vi "simulation de l ASSIETTE.vi"() -> ()   [LabVIEW 2016]
uses:
  <vilib>/Utility/miscctls.llb/LV3DPointTypeDef.ctl
  <vilib>/Instr/_visa.llb/VISA Configure Serial Port (Instr).vi
panel:
  in  "?":enum32{"Vue de l'ensemble"}(tab)
  out "2 2":dynamicdata(graph)
  in  "Aileron":dbl(slide) scale=-25.0..25.0
  out "Gimbal":refnum<vi>(3d-picture)
  in  "PITCH":dbl(slide) scale=-90.0..90.0
  in  "Profondeur":dbl(slide) scale=-35.0..35.0
  out "GAZ":dbl(slide) scale=0.0..35.0
  out "?":T1(graph)={"X"=[{"Y"=[21.620706805998168, 20.15124367946963, 12.465582235692763, 7.946576972490323, 11.656565240893995, 3.970903792227472, 5.440366929130449, 13.126028372052978, 19.003880895383112, 16.244982298473555, 16.832767550897515, 24.922937499080067, 24.33515224168201, 19.81289788882929, 13.93504536742159, 21.620706805998168], "Y"=[7.099604990531346, 5.077062500919932, 10.661022401488875, 5.291796067500631, 11.248807654089271, 16.832767550897515, 18.855310035128806, 13.271350139939326, 21.36152008350073, 25.220079209877188, 26.02909620777253, 20.151243679469633, 19.34222668734553, 20.773734831883043, 12.683564887248515, 7.099604990531346]}], "z"=[{"Y"=[15.0, 16.30733614, 17.60472267, 17.43107449, 17.60472267, 18.88228568, 20.13030215, 19.78828201, 20.13030215, 21.33927393, 22.5, 22.0, 22.5, 23.60364655, 24.64181415, 23.99902654, 24.64181415, 25.60660172, 26.49066665, 25.7246222, 26.49066665, 27.28728066, 27.99038106, 27.12435565, 27.99038106, 28.59461681, 29.09538931, 28.15569669, 29.09538931, 29.48888739, 29.7721163, 28.78730854, 29.7721163, 29.94292047, 30.0, 28.5, 30.0, 29.94292047, 29.7721163, 28.78730854, 29.7721163, 29.48888739, 29.09538931, 28.15569669, 29.09538931, 28.59461681, 27.99038106, 27.12435565, 27.99038106, 27.28728066, 26.49066665, 25.7246222, 26.49066665, 25.60660172, 24.64181415, 23.99902654, 24.64181415, 23.60364655, 22.5, 22.0, 22.5, 21.33927393, 20.13030215, 19.78828201, 20.13030215, 18.88228568, 17.60472267, 17.43107449, 17.60472267, 16.30733614, 15.0, 15.0, 15.0, 13.69266386, 12.39527733, 12.56892551, 12.39527733, 11.11771432, 9.86969785, 10.21171799, 9.86969785, 8.660726074, 7.5, 8.0, 7.5, 6.396353455, 5.358185855, 6.000973464, 5.358185855, 4.393398282, 3.509333353, 4.275377796, 3.509333353, 2.712719336, 2.009618943, 2.875644347, 2.009618943, 1.405383194, 0.904610688, 1.844303309, 0.904610688, 0.511112606, 0.227883705, 1.212691458, 0.227883705, 0.057079529, 0.0, 1.5, 0.0, 0.057079529, 0.227883705, 1.212691458, 0.227883705, 0.511112606, 0.904610688, 1.844303309, 0.904610688, 1.405383194, 2.009618943, 2.875644347, 2.009618943, 2.712719336, 3.509333353, 4.275377796, 3.509333353, 4.393398282, 5.358185855, 6.000973464, 5.358185855, 6.396353455, 7.5, 8.0, 7.5, 8.660726074, 9.86969785, 10.21171799, 9.86969785, 11.11771432, 12.39527733, 12.56892551, 12.39527733, 13.69266386, 15.0, 15.0], "Y"=[30.0, 29.94292047, 29.7721163, 28.78730854, 29.7721163, 29.48888739, 29.09538931, 28.15569669, 29.09538931, 28.59461681, 27.99038106, 27.12435565, 27.99038106, 27.28728066, 26.49066665, 25.7246222, 26.49066665, 25.60660172, 24.64181415, 23.99902654, 24.64181415, 23.60364655, 22.5, 22.0, 22.5, 21.33927393, 20.13030215, 19.78828201, 20.13030215, 18.88228568, 17.60472267, 17.43107449, 17.60472267, 16.30733614, 15.0, 15.0, 15.0, 13.69266386, 12.39527733, 12.56892551, 12.39527733, 11.11771432, 9.86969785, 10.21171799, 9.86969785, 8.660726074, 7.5, 8.0, 7.5, 6.396353455, 5.358185855, 6.000973464, 5.358185855, 4.393398282, 3.509333353, 4.275377796, 3.509333353, 2.712719336, 2.009618943, 2.875644347, 2.009618943, 1.405383194, 0.904610688, 1.844303309, 0.904610688, 0.511112606, 0.227883705, 1.212691458, 0.227883705, 0.057079529, 0.0, 1.5, 0.0, 0.057079529, 0.227883705, 1.212691458, 0.227883705, 0.511112606, 0.904610688, 1.844303309, 0.904610688, 1.405383194, 2.009618943, 2.875644347, 2.009618943, 2.712719336, 3.509333353, 4.275377796, 3.509333353, 4.393398282, 5.358185855, 6.000973464, 5.358185855, 6.396353455, 7.5, 8.0, 7.5, 8.660726074, 9.86969785, 10.21171799, 9.86969785, 11.11771432, 12.39527733, 12.56892551, 12.39527733, 13.69266386, 15.0, 15.0, 15.0, 16.30733614, 17.60472267, 17.43107449, 17.60472267, 18.88228568, 20.13030215, 19.78828201, 20.13030215, 21.33927393, 22.5, 22.0, 22.5, 23.60364655, 24.64181415, 23.99902654, 24.64181415, 25.60660172, 26.49066665, 25.7246222, 26.49066665, 27.28728066, 27.99038106, 27.12435565, 27.99038106, 28.59461681, 29.09538931, 28.15569669, 29.09538931, 29.48888739, 29.7721163, 28.78730854, 29.7721163, 29.94292047, 30.0, 28.5]}]}
  in  "ROLL":dbl(slide) scale=-90.0..90.0
  in  "Directions":dbl(slide) scale=-25.0..25.0
  in  "visual":refnum<k7>(container) caption="3D 파라미터형 표면"
  out "2":dynamicdata(graph)
  out "Temperature":dbl caption="degC" format="%.1f"
  out "Altitude Estimée":dbl caption="m" format="%.1f"
  in  "VISA resource name":refnum<visa-resource-name>
  in  "yaw":dbl(slide) scale=0.0..360.0
  in  "stop":bool
  in  "Heading":dbl(knob) scale=-360.0..360.0
  out "?":timestamp
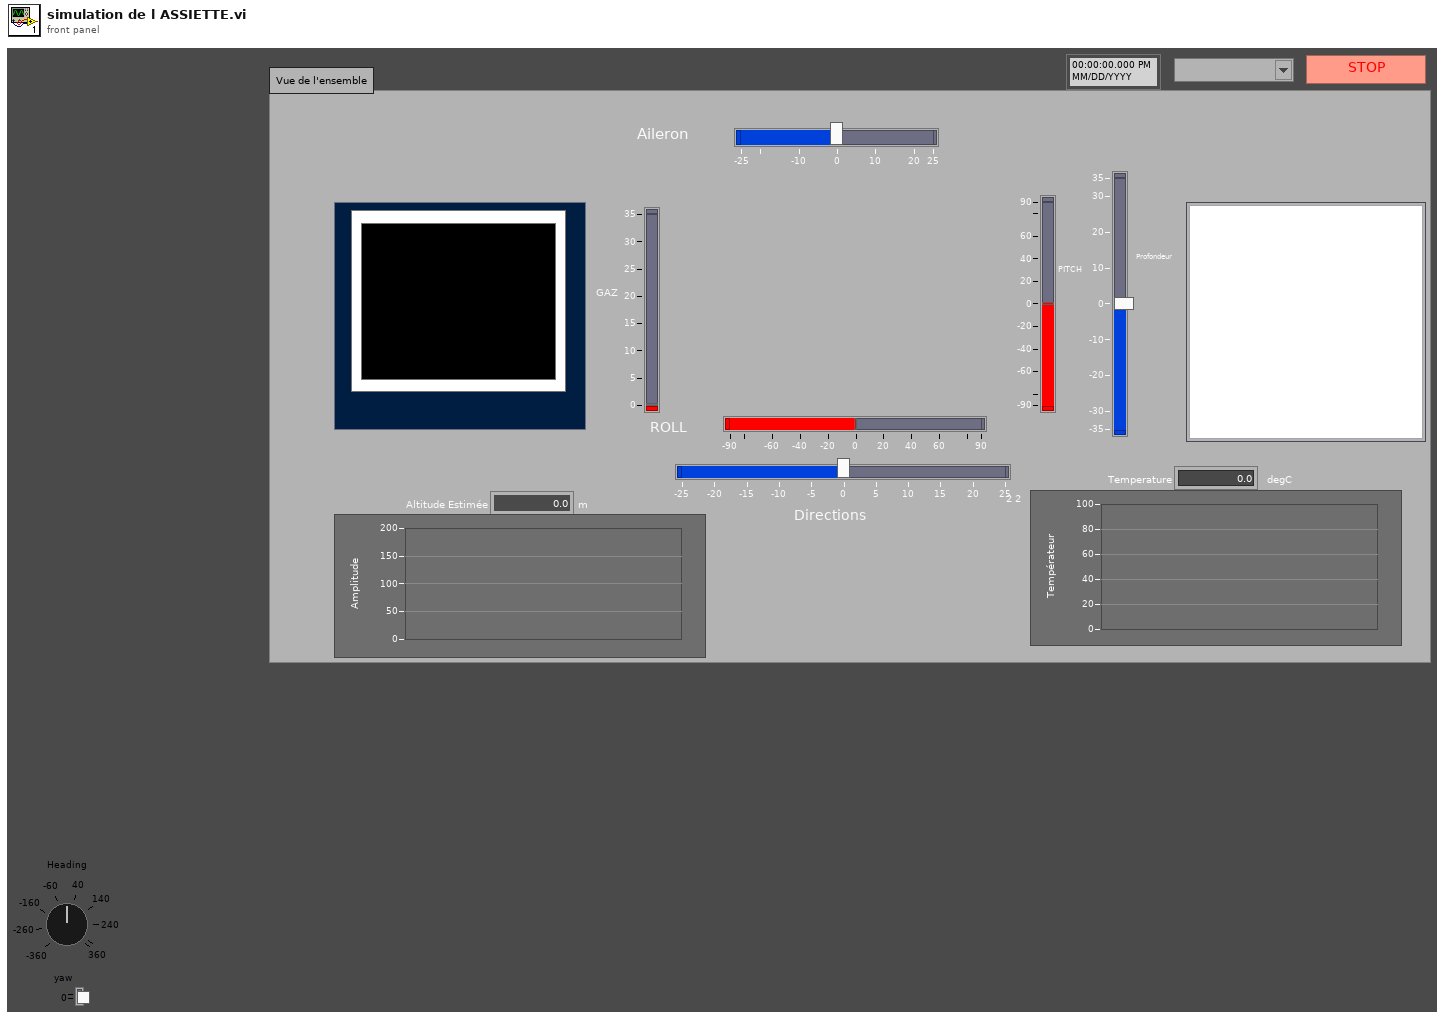
[diagram p1: front panel]
types:
  T1 = cluster{"X":cluster{"Y":dbl[], "Y":dbl[]}[], "z":cluster{"Y":dbl[], "Y":dbl[]}[]}
  T2 = typedef "gimbal data.ctl" = cluster{"Dial Ref":refnum<vi>, "Drum Ref":refnum<vi>, "Window Ref":refnum<vi>, "First Scene":refnum<vi>, "last pitch":dbl, "last roll":dbl, "last dial":dbl}
  T3 = typedef "LV3DPointTypeDef.ctl" = cluster{"X":sgl, "Y":sgl, "Z":sgl}
  T4 = cluster{"Aircraft":cluster{"Y":dbl[], "Y":dbl[]}[], "Circle":cluster{"Y":dbl[], "Y":dbl[]}[]}
  T5 = cluster{"[0]":dbl, "[Aileron]":dbl, "[profondeur]":dbl, "[dirction]":dbl, "[gaz]":dbl, "[5]":dbl, "[6]":dbl, "[7]":dbl, "[8]":dbl}
  T6 = cluster{"[0]":dbl, "[yaw]":dbl, "[pitch]":dbl, "[roll]":dbl, "[heading]":dbl, "[temp]":dbl, "[altitue]":dbl, "[7]":dbl, "[8]":dbl}
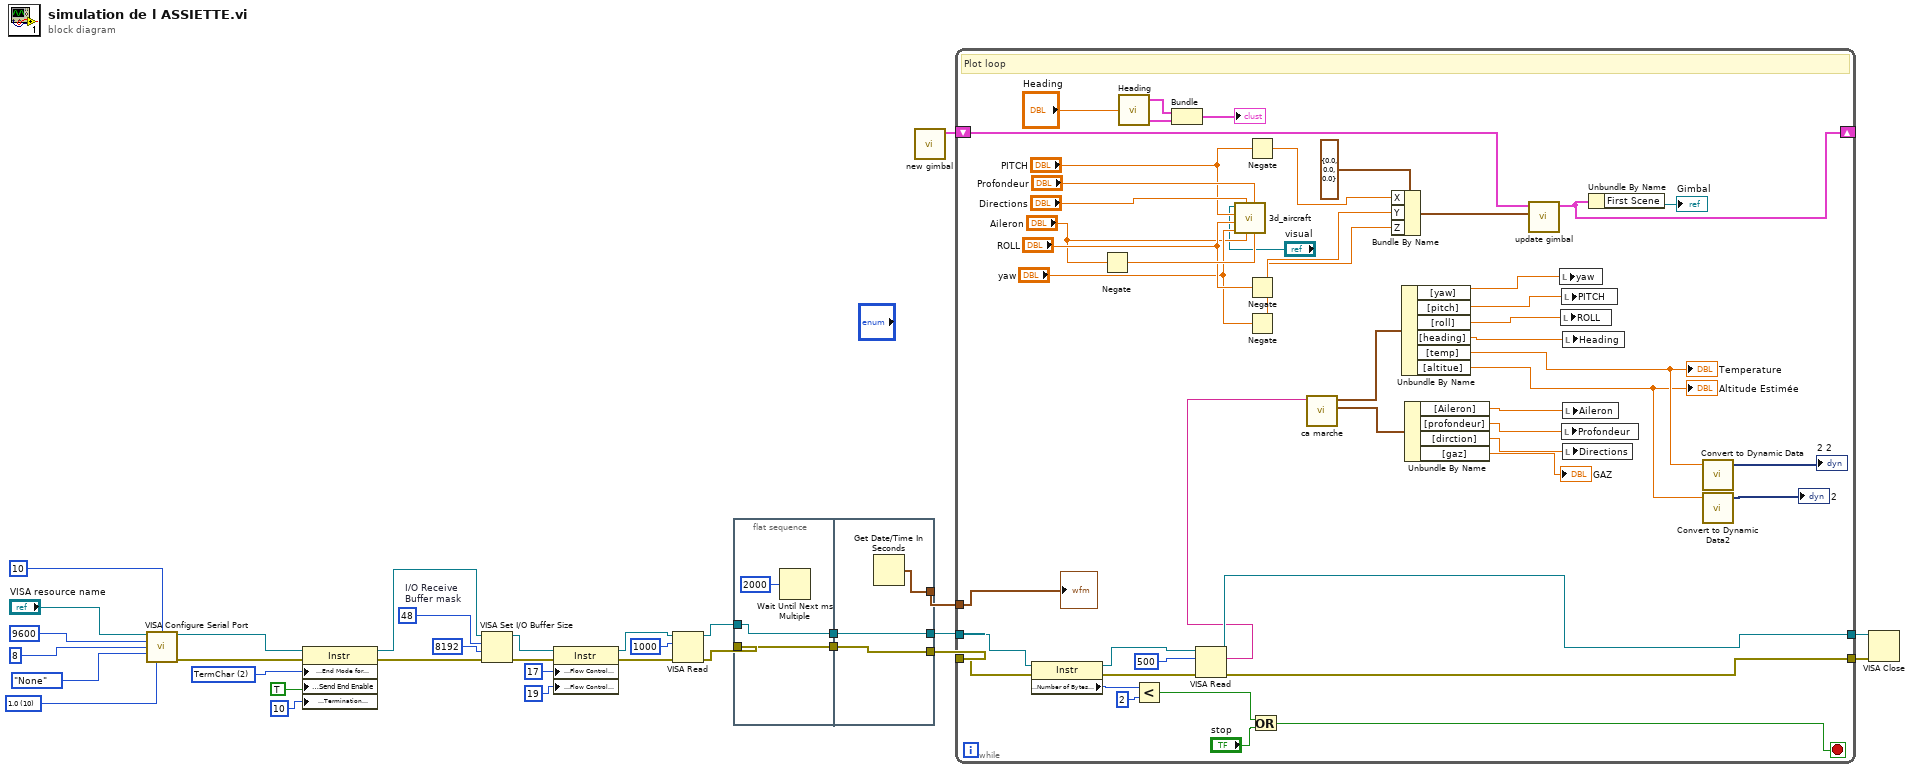
[diagram p0: block diagram]
diagram:
  w10 = u16 10 items=["1.0"=10, "1.5"=15, "2.0"=20] ("stop bits (10: 1 bit)")
  w27 = u16 48  # I/O Receive Buffer mask
  w16 = u16 2 items=["None", "LastBit", "TermChar", "Break"] ("Serial Settings:Serial End Mode for Writes")
  n1 = call-poly "VISA Configure Serial Port"("VISA resource name"="VISA resource name", "termination char\n(0xA = '\\n' = LF)"=u8 10 ("termination char\n(0xA = '\\n' = LF)"), "baud rate (9600)"=u32 9600, "data bits (8)"=u16 8, "parity (0:none)"=enum16{"None", "Odd", "Even", "Mark", "Space"}."None", "stop bits (10: 1 bit)"=w10) -> ("VISA resource name out"=w7:refnum<visa-resource-name>, "error out"=w6:errorcluster)  [unwired: 8 in]
  n2 = property class="Instr"(reference=w7, error in=w6, "Serial Settings:End Mode for Writes"=w16, "Message Based Settings:Send End Enable"=TRUE, "Message Based Settings:Termination Character"=u8 10 ("termination char\n(0xA = '\\n' = LF)")) -> (reference out=w25:refnum<visa-resource-name>, error out=w19:errorcluster)
  n3 = VISA Set I/O Buffer Size(VISA resource name=w25, mask (16)=w27, size (4096)=u32 8192 ("Input\nbuffer size"), error in (no error)=w19) -> (VISA resource name out=w22:refnum<visa-resource-name>, error out=w18:errorcluster)
  n4 = property class="Instr"(reference=w22, error in=w18, "Serial Settings:Flow Control XON Character"=u8 17 ("XON Character"), "Serial Settings:Flow Control XOFF Character"=u8 19 ("XOFF Character")) -> (reference out=w21:refnum<visa-resource-name>, error out=w17:errorcluster)
  n5 = VISA Read(VISA resource name=w21, byte count=u32 1000, error in (no error)=w17) -> (VISA resource name out=w1:refnum<visa-resource-name>, error out=w2:errorcluster)  [unwired: 2 out]
  n6 = flat-sequence {
    tunnel: w2 -> [w35]
    tunnel: [w35] -> w32
    tunnel: w1 -> [w34]
    tunnel: [w34] -> w31
    tunnel: [w36] -> w5
    tunnel: [w38] -> w4
    tunnel: [w37] -> w3
    tunnel: w32 -> [w38]
    tunnel: w31 -> [w36]
    frame #0 {
      n7 = Wait Until Next ms Multiple(millisecond multiple=u32 2000 ("n millisecondes")) -> ()  [unwired: 1 out]
    }
    frame #1 {
      n8 = Get Date/Time In Seconds() -> (seconds since 1Jan1904=w37:timestamp)
    }
  }
  n9 = call "new gimbal.vi"() -> ("Data"=w30:T2)  [unwired: 10 in, 1 out]
  n10 = while {
    shift-right: [w83] -> _
    shift-left: w30 -> [w84]
    tunnel: w4 -> [w61]
    tunnel: w5 -> [w62]
    tunnel: [w56] -> w15
    tunnel: [w60] -> w14
    tunnel: w3 -> [w52]
    stop <- w58 stop-if-true
    # "Plot loop"
    n11 = property class="Instr"(reference=w62, error in=w61) -> (reference out=w66:refnum<visa-resource-name>, error out=w65:errorcluster, "Serial Settings:Number of Bytes at Serial Port"=w64:u32)
    n12 = Negate(x="Aileron") -> (-x=w86:dbl)
    n13 = call "Heading.vi"("각도"="Heading") -> ("Circle"=w71:cluster{"Y":dbl[], "Y":dbl[]}[], "Aircraft"=w69:cluster{"Y":dbl[], "Y":dbl[]}[])  [unwired: 3 in]
    n14 = Less?(x=w64, y=u32 2) -> (x < y?=w59:bool)
    n15 = Bundle("Aircraft"=w69, "Circle"=w71) -> (→"?":T4)  [unwired: 1 in]
    n16 = VISA Read(VISA resource name=w66, byte count=u32 500, error in (no error)=w65) -> (VISA resource name out=w56:refnum<visa-resource-name>, read buffer=w51:string, error out=w60:errorcluster)  [unwired: 1 out]
    n17 = call "3d_aircraft.vi"("RH Aileron"=w86, "Elevator"="Profondeur", "LH Aileron"="Aileron", "Rudder"="Directions", "Heading (deg)"="yaw", "Roll (deg)"="ROLL", "Pitch (deg)"="PITCH", "visual"="visual") -> ()  [unwired: 4 in]
    n18 = Negate(x="PITCH") -> (-x=w80:dbl)
    n19 = Negate(x="ROLL") -> (-x=w79:dbl)
    n20 = Negate(x="yaw") -> (-x=w78:dbl)
    n21 = Or(x=w59, y="stop") -> (x .or. y?=w58:bool)
    n22 = call "ca marche.vi"("chaîne de type tableur"=w51) -> ("cluster"=w43:T5, 3:w50:T6)  [unwired: 9 in]
    n23 = Bundle By Name(cluster=T3 {"X"=0.0, "Y"=0.0, "Z"=0.0} ("Control 1"), "X"=w80, "Y"=w79, "Z"=w78) -> (w81:T3)
    n24 = Unbundle By Name(w50) -> ("[yaw]"=w49:dbl, "[pitch]"=w48:dbl, "[roll]"=w47:dbl, "[heading]"=w46:dbl, "[temp]"=w45:dbl, "[altitue]"=w44:dbl)
    "Temperature" <- w45
    "Altitude Estimée" <- w44
    n25 = Unbundle By Name(w43) -> ("[Aileron]"=w42:dbl, "[profondeur]"=w41:dbl, "[dirction]"=w40:dbl, "[gaz]"=→"GAZ":dbl)
    n26 = call "update gimbal.vi"("Current Position"=w81, "Data"=w84) -> ("Data"=w83:T2)  [unwired: 8 in, 1 out]
    n27 = local write "yaw"(w49) -> ()
    n28 = local write "ROLL"(w47) -> ()
    n29 = local write "PITCH"(w48) -> ()
    n30 = local write "Profondeur"(w41) -> ()
    n31 = local write "Heading"(w46) -> ()
    n32 = local write "Aileron"(w42) -> ()
    n33 = local write "Directions"(w40) -> ()
    n34 = Unbundle By Name(w83) -> ("First Scene"=→"Gimbal":refnum<vi>)
    n35 = call "Convert to Dynamic Data"("Double"=w45) -> ("Dynamic Data Type"=→"2 2":dynamicdata)  [unwired: 3 in]
    n36 = call "Convert to Dynamic Data2"("Double"=w44) -> ("Dynamic Data Type"=→"2":dynamicdata)  [unwired: 3 in]
    "?" <- w52
  }
  n37 = VISA Close(VISA resource name=w15, error in (no error)=w14) -> ()  [unwired: 1 out]
